vi "9219_UpdateConfigControls.vi"(0 "_Decorations":T2, 4 "RTD Refnum":refnum<vi>, 5 "CVD Refs":refnum<vi>[](array[refnum]), 6 "Range2 Refnum":refnum<vi>, 8 "Threshold Refnum":refnum<vi>, 9 "Range Refnum":refnum<vi>, 10 "Selected Channels":i32[](array[numeric]), 11 "9219 Config":T1 {"Conversion Time" items=["High Speed", "Best 60 Hz Rejection", "Best 50 Hz Rejection", "High Resolution"]; "TCoupleType" items=["J", "K", "T", "E", "R", "S", "N", "B"]; "DegreeRange" items=["Raw units", "Degrees Kelvin", "Degrees Celsius", "Degrees Fahrenheit", "Degrees Rankine"]; "RtdType" items=["TCR3851"=1, "TCR3750"=2, "TCR3916"=3, "TCR3920"=4, "TCR3911"=5, "TCR3928"=6, "Custom"=0]}) -> (2 "Mode value":u8, 3 "Valid mode?":bool)   [LabVIEW 2017, in "Modules.lvlib" / "9219.lvclass"]
uses:
  9219.lvclass
  9219 Config.ctl
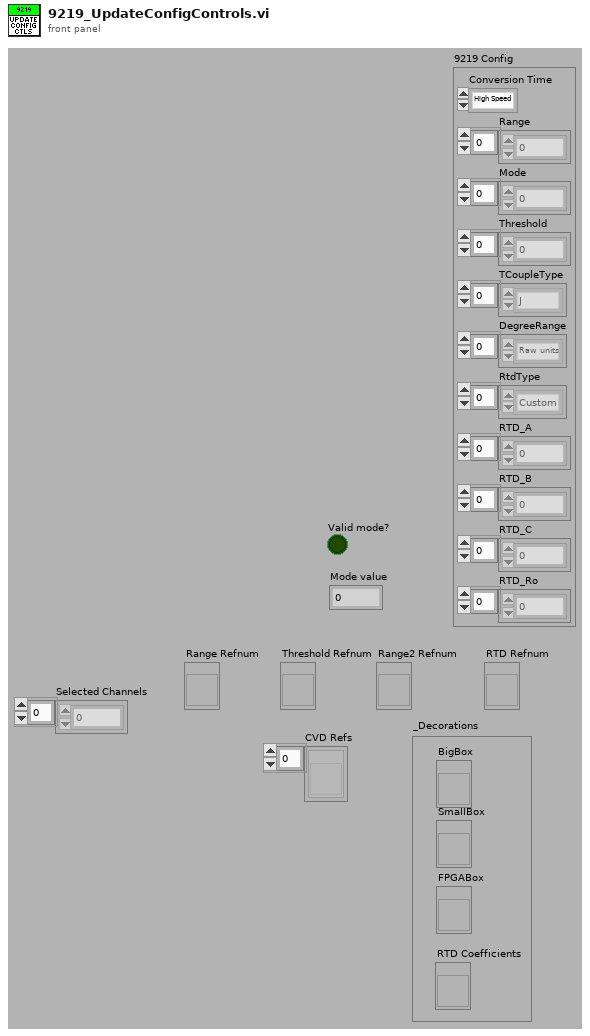
[diagram p1: front panel]
types:
  T1 = typedef "Modules.lvlib/9219.lvclass/9219 Config.ctl" = cluster{"Conversion Time":u16, "Range":u8[], "Mode":u8[], "Threshold":dbl[], "TCoupleType":u8[], "DegreeRange":u8[], "RtdType":u8[], "RTD_A":dbl[], "RTD_B":dbl[], "RTD_C":dbl[], "RTD_Ro":dbl[]}
  T2 = cluster{"SmallBox":refnum<vi>, "BigBox":refnum<vi>, "FPGABox":refnum<vi>, "RTD Coefficients":refnum<vi>}
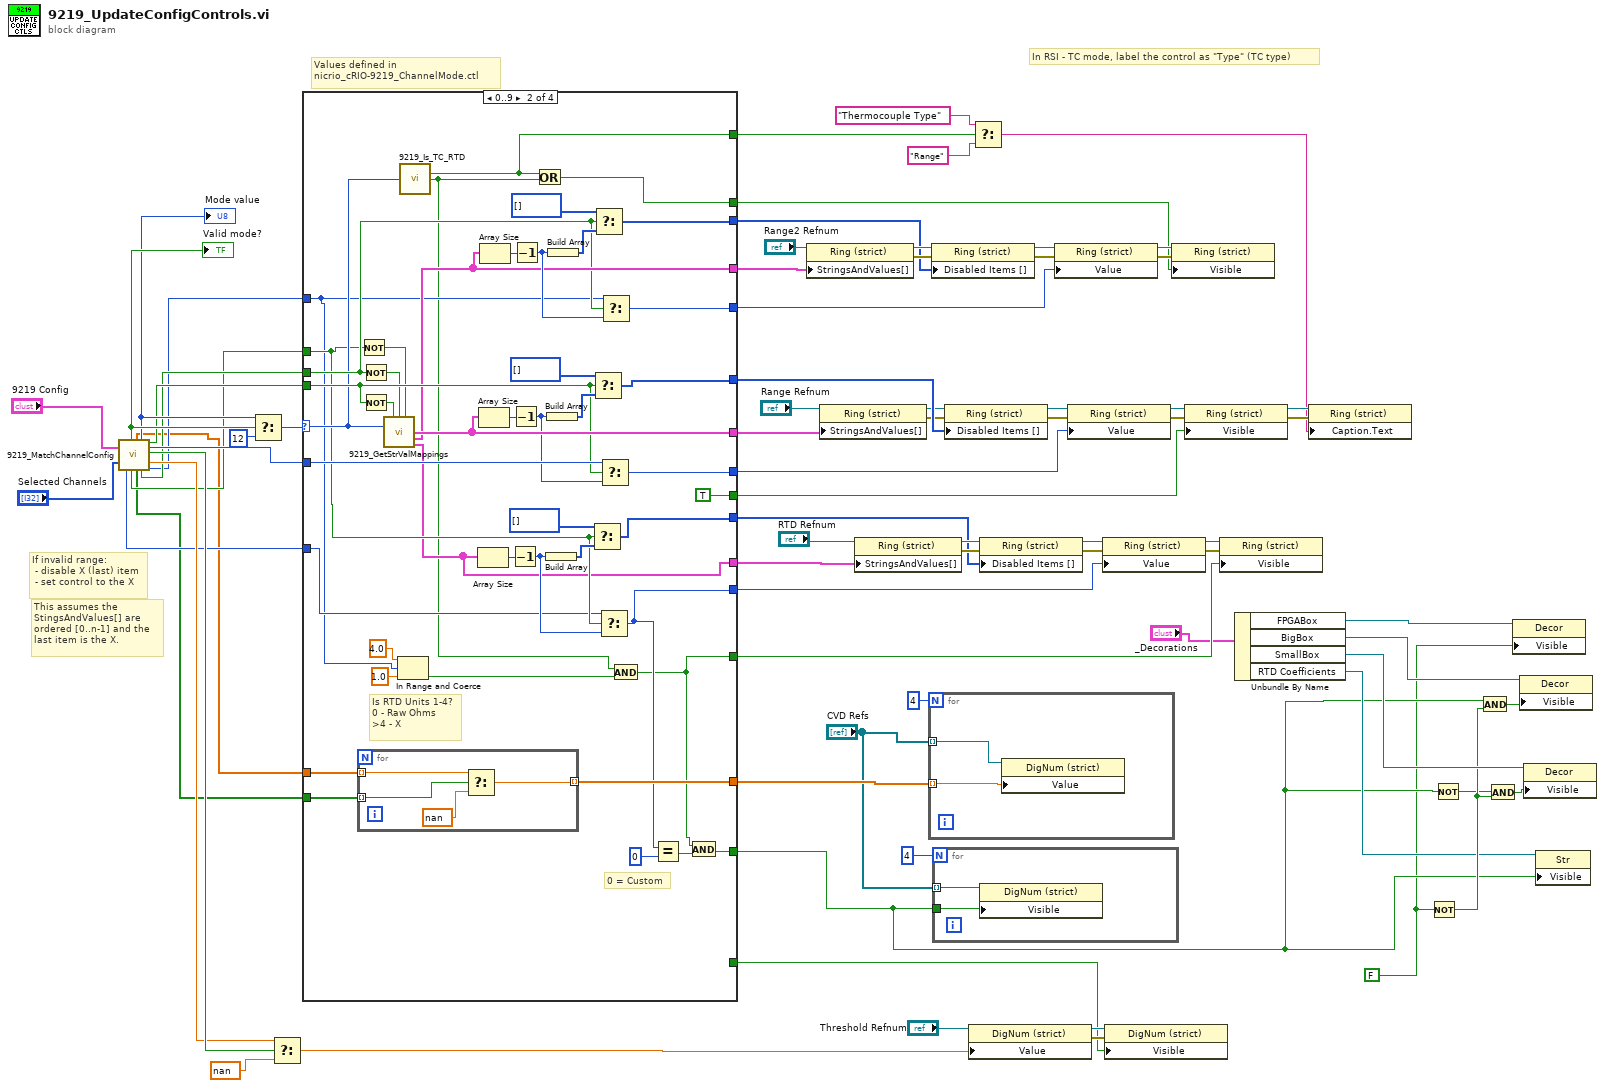
[diagram p0: block diagram]
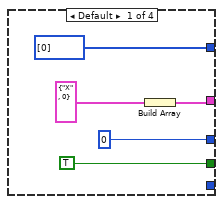
[diagram p2: hidden frame]
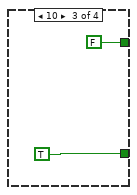
[diagram p3: hidden frame]
diagram:
  w3 = FALSE
  # "This assumes the StingsAndValues[] are ordered [0..n-1] and the last item is the X."
  # "If invalid range:\n - disable X (last) item\n - set control to the X"
  # "In RSI - TC mode, label the control as \"Type\" (TC type)"
  # "Values defined in \nnicrio_cRIO-9219_ChannelMode.ctl"
  n1 = call "9219_MatchChannelConfig.vi"("ConfigTD in"="9219 Config", "Selected Channels"="Selected Channels") -> ("Type RTD"=w30:u8, "Valid mode?"=w54:bool, "Valid RTD?"=w31:bool, "CVD"=w21:dbl[], "Vald CVD"=w20:bool[], "Mode value"=w53:u8, "Valid range2?"=w48:bool, "Valid range?"=w52:bool, "Range value"=w49:u8, "Valid threshold?"=w51:bool, "Threshold value"=w50:dbl, "Type range2"=w47:u8)  [unwired: 6 in]
  "Valid mode?" <- w54
  "Mode value" <- w53
  n2 = Select(t=w53, s=w54, f=12 ("t")) -> (s? t:f=w66:i32)
  n3 = Select(t=w50, s=w51, f=nan ("t")) -> (s? t:f=w65:dbl)
  n4 = case shown="0..9" w66 {
    selector: w66 -> [_ w100 _ _]
    tunnel: [w72 w116 _ _] -> w70
    tunnel: [0 ("Value1") w120 _ _] -> w69
    tunnel: w52 -> [_ w114 _ _]
    tunnel: [i32[] [0] ("Disabled Items []") w117 _ _] -> w67
    tunnel: [TRUE ("Visible") TRUE ("Visible") _ _] -> w68
    tunnel: [_ _ TRUE ("Visible") _] -> w45
    tunnel: w49 -> [_ w119 _ _]
    tunnel: w48 -> [_ w103 _ _]
    tunnel: w47 -> [_ w81 _ _]
    tunnel: [_ w104 _ _] -> w39
    tunnel: [_ w102 _ _] -> w38
    tunnel: [_ w101 _ _] -> w37
    tunnel: [_ w99 _ _] -> w32
    tunnel: [_ w98 _ _] -> w34
    tunnel: w31 -> [_ w92 _ _]
    tunnel: w30 -> [_ w91 _ _]
    tunnel: [_ w90 _ _] -> w24
    tunnel: [_ w85 _ _] -> w23
    tunnel: [_ w89 _ _] -> w22
    tunnel: [_ w76 _ _] -> w15
    tunnel: w21 -> [_ w88 _ _]
    tunnel: w20 -> [_ w87 _ _]
    tunnel: [_ w86 _ _] -> w19
    tunnel: [_ w78 FALSE _] -> w5
    frame Default {
      n5 = Build Array(cluster{"String":string, "Value":u16} {"String"="X", "Value"=0}) -> (w72:cluster{"String":string, "Value":u16}[])
    }
    frame 0..9 {
      # "Is RTD Units 1-4?\n0 - Raw Ohms\n>4 - X"
      # "0 = Custom"
      n6 = for {
        tunnel: w88 -> [w123] mode=indexing
        tunnel: w87 -> [w124] mode=indexing
        tunnel: [w121] -> w86 mode=indexing
        n7 = Select(t=w123, s=w124, f=nan) -> (s? t:f=w121:dbl)
      }
      n8 = Not(x=w92) -> (.not. x?=w93:bool)
      n9 = Not(x=w103) -> (.not. x?=w110:bool)
      n10 = Not(x=w114) -> (.not. x?=w113:bool)
      n11 = call "9219_GetStrValMappings.vi"("_Include \"invalid\" Range item (F)"=w113, "_Include \"invalid\" Range2 item (F)"=w110, "_Include \"invalid\" RTD (F)"=w93, "_Mode"=w100) -> ("_Range Strings And Values []"=w116:cluster{"String":string, "Value":u16}[], "_Range2 Strings And Values []"=w104:cluster{"String":string, "Value":u16}[], "_RTD Strings And Values []"=w89:cluster{"String":string, "Value":u16}[])  [unwired: 8 in, 1 out]
      n12 = In Range and Coerce(upper limit=4.0, x=w81, lower limit=1.0) -> (In Range?=w77:bool)  [unwired: 1 out]
      n13 = call "9219_Is_TC_RTD.vi"("Mode"=w100) -> ("Is RIOScan / Thermocouple"=w98:bool, "Is RIOScan / RTD"=w80:bool)  [unwired: 13 in]
      n14 = Array Size(array=w89) -> (size(s)=w96:i32)
      n15 = Array Size(array=w116) -> (size(s)=w112:i32)
      n16 = Array Size(array=w104) -> (size(s)=w107:i32)
      n17 = Decrement(x=w96) -> (x-1=w97:i32)
      n18 = Decrement(x=w112) -> (x-1=w111:i32)
      n19 = Decrement(x=w107) -> (x-1=w108:i32)
      n20 = Or(x=w98, y=w80) -> (x .or. y?=w99:bool)
      n21 = Build Array(w97) -> (w95:i32[])
      n22 = Build Array(w111) -> (w115:i32[])
      n23 = Build Array(w108) -> (w106:i32[])
      n24 = Select(t=i32[] [], s=w92, f=w95) -> (s? t:f=w90:i32[])
      n25 = Select(t=i32[] [], s=w114, f=w115) -> (s? t:f=w117:i32[])
      n26 = Select(t=i32[] [], s=w103, f=w106) -> (s? t:f=w101:i32[])
      n27 = Select(t=w91, s=w92, f=w97) -> (s? t:f=w85:i32)
      n28 = Select(t=w119, s=w114, f=w111) -> (s? t:f=w120:i32)
      n29 = Select(t=w81, s=w103, f=w108) -> (s? t:f=w102:i32)
      n30 = And(x=w80, y=w77) -> (x .and. y?=w76:bool)
      n31 = Equal?(x=w85, y=0) -> (x = y?=w79:bool)
      n32 = And(x=w76, y=w79) -> (x .and. y?=w78:bool)
    }
    frame 10 {
    }
    frame 11 {
    }
  }
  n33 = property on="Property Node" class="Ring (strict)"(reference="Range2 Refnum", "StringsAndValues[]"=w39) -> (error out=w41:errorcluster)  [unwired: 1 in, 1 out]
  n34 = property on="Property Node" class="Ring (strict)"(reference="Range Refnum", "StringsAndValues[]"=w70) -> (error out=w61:errorcluster)  [unwired: 1 in, 1 out]
  n35 = property on="Property Node" class="Ring (strict)"(reference="RTD Refnum", "StringsAndValues[]"=w22) -> (error out=w26:errorcluster)  [unwired: 1 in, 1 out]
  n36 = for {
    N: 4 -> [_]
    tunnel: "CVD Refs" -> [w128] mode=indexing
    tunnel: w19 -> [w127] mode=indexing
    n37 = property on="Property Node" class="DigNum (strict)"(reference=w128, "Value"=w127) -> ()  [unwired: 1 in, 2 out]
  }
  n38 = property on="Property Node" class="Ring (strict)"(reference="Range2 Refnum", error in=w41, "Disabled Items []"=w37) -> (error out=w42:errorcluster)  [unwired: 1 out]
  n39 = for {
    N: 4 -> [_]
    tunnel: w5 -> [w130]
    tunnel: "CVD Refs" -> [w129] mode=indexing
    n40 = property on="Property Node" class="DigNum (strict)"(reference=w129, "Visible"=w130) -> ()  [unwired: 1 in, 2 out]
  }
  n41 = property on="Property Node" class="Ring (strict)"(reference="Range Refnum", error in=w61, "Disabled Items []"=w67) -> (error out=w60:errorcluster)  [unwired: 1 out]
  n42 = property on="Property Node" class="DigNum (strict)"(reference="Threshold Refnum", "Value"=w65) -> (reference out=w56:refnum<vi>, error out=w57:errorcluster)  [unwired: 1 in]
  n43 = Select(t="Thermocouple Type" ("Section"), s=w34, f="Range" ("String ID")) -> (s? t:f=w33:string)
  n44 = property on="Property Node" class="Ring (strict)"(reference="RTD Refnum", error in=w26, "Disabled Items []"=w24) -> (error out=w27:errorcluster)  [unwired: 1 out]
  n45 = property on="Property Node" class="Ring (strict)"(reference="Range2 Refnum", error in=w42, "Value"=w38) -> (reference out=w44:refnum<vi>, error out=w43:errorcluster)
  n46 = property on="Property Node" class="Ring (strict)"(reference="Range Refnum", error in=w60, "Value"=w69) -> (reference out=w58:refnum<vi>, error out=w59:errorcluster)
  n47 = property on="Property Node" class="Ring (strict)"(reference="RTD Refnum", error in=w27, "Value"=w23) -> (reference out=w29:refnum<vi>, error out=w28:errorcluster)
  n48 = property on="Property Node" class="DigNum (strict)"(reference=w56, error in=w57, "Visible"=w45) -> ()  [unwired: 2 out]
  n49 = property on="Property Node" class="Ring (strict)"(reference=w44, error in=w43, "Visible"=w32) -> ()  [unwired: 2 out]
  n50 = property on="Property Node" class="Ring (strict)"(reference=w58, error in=w59, "Visible"=w68) -> (reference out=w36:refnum<vi>, error out=w35:errorcluster)
  n51 = property on="Property Node" class="Ring (strict)"(reference=w29, error in=w28, "Visible"=w15) -> ()  [unwired: 2 out]
  n52 = Unbundle By Name("_Decorations") -> ("FPGABox"=w12:refnum<vi>, "BigBox"=w14:refnum<vi>, "SmallBox"=w13:refnum<vi>, "RTD Coefficients"=w6:refnum<vi>)
  n53 = property on="Property Node" class="Ring (strict)"(reference=w36, error in=w35, "Caption.Text"=w33) -> ()  [unwired: 2 out]
  n54 = Not(x=w3) -> (.not. x?=w9:bool)
  n55 = Not(x=w5) -> (.not. x?=w8:bool)
  n56 = And(x=w5, y=w9) -> (x .and. y?=w11:bool)
  n57 = And(x=w8, y=w9) -> (x .and. y?=w10:bool)
  n58 = property class="Decor"(reference=w12, "Visible"=w3) -> ()  [unwired: 1 in, 2 out]
  n59 = property class="Decor"(reference=w14, "Visible"=w11) -> ()  [unwired: 1 in, 2 out]
  n60 = property class="Decor"(reference=w13, "Visible"=w10) -> ()  [unwired: 1 in, 2 out]
  n61 = property on="Property Node" class="Str"(reference=w6, "Visible"=w5) -> ()  [unwired: 1 in, 2 out]
